vi "Sig_AI_Create.vi"(0 "reference in":refnum<class "Sig_AI.lvclass">, 5 "error in (no error)":errorcluster) -> (14 "reference out":refnum<class "Sig_AI.lvclass">, 19 "error out":errorcluster)   [LabVIEW 2019, in "Sig_AI.lvclass"]
doc: "Constructor."
uses:
  Sig_AI.lvclass
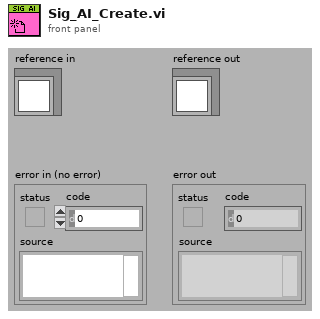
[diagram p1: front panel]
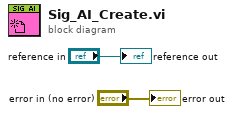
[diagram p0: block diagram]
diagram:
  "error out" <- "error in (no error)"
  "reference out" <- "reference in"
